vi "OPM.SetWavelength.vi"(8 "error in (no error)":errorcluster, 10 "Wavelength, nm":dbl, 11 "OPM in":refnum<class "OPM.lvclass">) -> (0 "error out":errorcluster, 3 "OPM out":refnum<class "OPM.lvclass">)   [LabVIEW 2019, in "OPM.lvclass"]
uses:
  OPM.lvclass
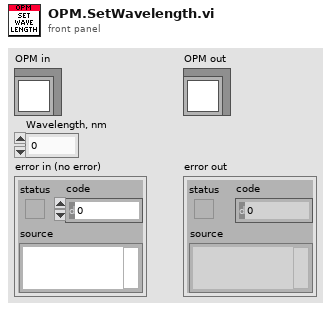
[diagram p1: front panel]
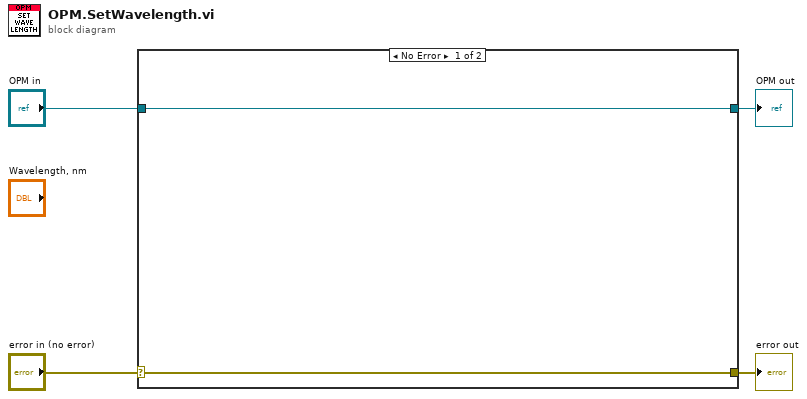
[diagram p0: block diagram]
diagram:
  n1 = case shown="No Error" "error in (no error)" {
    selector: "error in (no error)" -> [w5 w8]
    tunnel: [w5 w8] -> w3
    tunnel: [w6 w7] -> w1
    tunnel: "OPM in" -> [w6 w7]
    frame No Error {
    }
    frame Error {
    }
  }
  "error out" <- w3
  "OPM out" <- w1
